vi "control.vi"(0 "tiempo (ms)":dbl, 5 "opticalPathMax (nm)":dbl, 7 "#samples":u32, 9 "lamda (nm)":dbl, 10 "SigmaMax (ms)":dbl, 12 "m":dbl, 13 "b":dbl) -> ()   [LabVIEW 2010]
panel:
  out "Prueba":dbl[](array[numeric])
  out "Final":dbl[](array[numeric])
  in  "queda?":bool=TRUE
  in  "delta t0 (ms)":dbl
  in  "Contraste":i32
  in  "Control?":bool
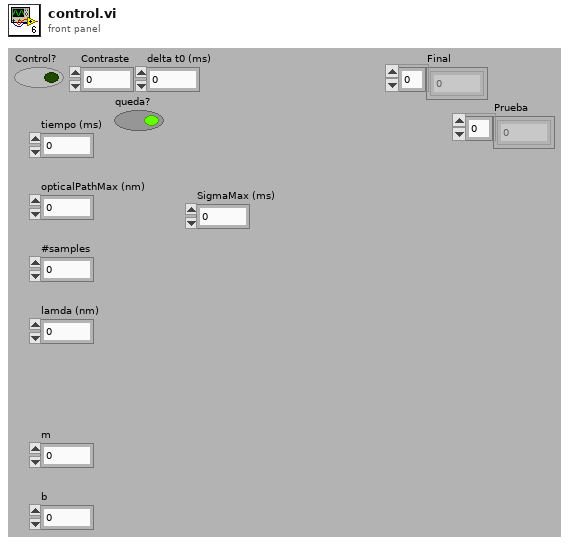
[diagram p1: front panel]
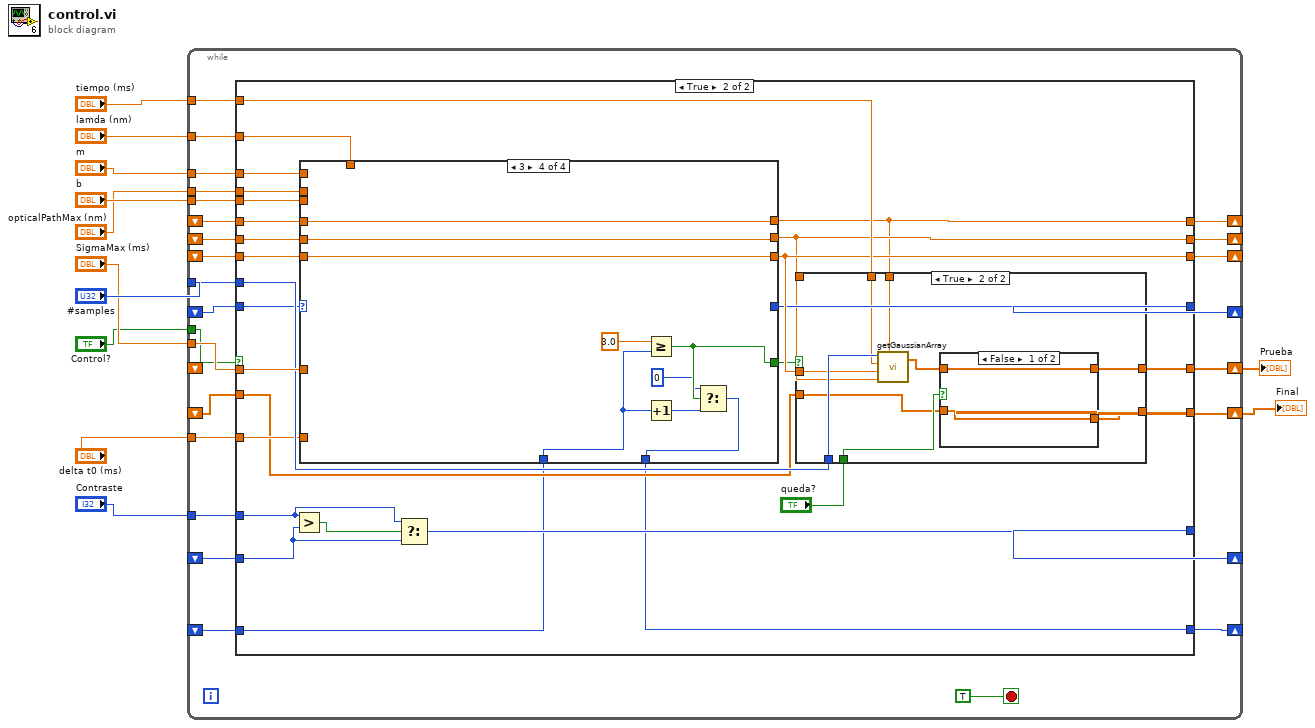
[diagram p0: block diagram]
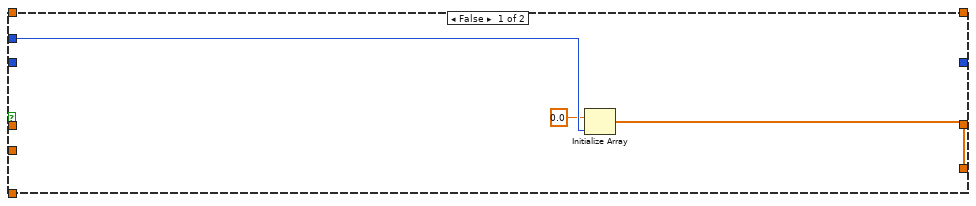
[diagram p2: hidden frame]
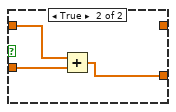
[diagram p4: hidden frame]
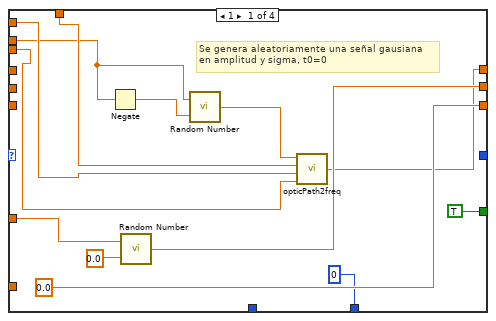
[diagram p5: hidden frame]
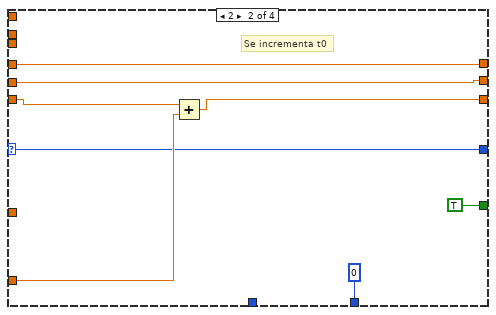
[diagram p6: hidden frame]
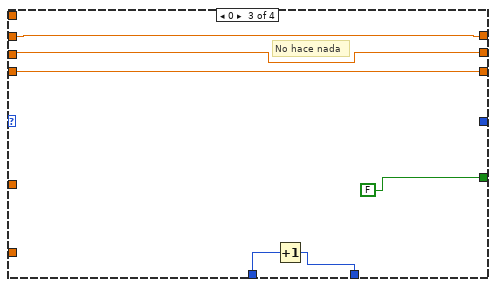
[diagram p7: hidden frame]
diagram:
  n1 = while {
    tunnel: "#samples" -> [w32]
    tunnel: "tiempo (ms)" -> [w31]
    shift-right: [w28] -> _
    shift-left: _ -> [w23]
    shift-right: [w29] -> _
    shift-left: _ -> [w22]
    shift-right: [w30] -> _
    shift-left: _ -> [w21]
    shift-right: [w17] -> _
    shift-left: _ -> [w18]
    tunnel: "lamda (nm)" -> [w37]
    tunnel: "m" -> [w36]
    tunnel: "b" -> [w35]
    tunnel: "SigmaMax (ms)" -> [w34]
    tunnel: "opticalPathMax (nm)" -> [w33]
    tunnel: "Contraste" -> [w26]
    shift-right: [w24] -> _
    shift-left: _ -> [w25]
    tunnel: "delta t0 (ms)" -> [w20]
    tunnel: "Control?" -> [w19]
    shift-right: [w27] -> w2
    shift-left: _ -> [w16]
    shift-right: [w15] -> w1
    shift-left: _ -> [_]
    shift-right: [w13] -> _
    shift-left: _ -> [w14]
    stop <- TRUE stop-if-true
    n2 = case shown="True" w19 {
      tunnel: w37 -> [_ w68]
      tunnel: w36 -> [_ w67]
      tunnel: w35 -> [_ w66]
      tunnel: w34 -> [_ w65]
      tunnel: w33 -> [_ w64]
      tunnel: w32 -> [w40 w63]
      tunnel: w31 -> [_ w62]
      tunnel: [_ w61] -> w30
      tunnel: [_ w60] -> w29
      tunnel: [_ w59] -> w28
      tunnel: [w41 w48] -> w27
      tunnel: w26 -> [_ w57]
      tunnel: w25 -> [_ w56]
      tunnel: [_ w55] -> w24
      tunnel: w23 -> [_ w54]
      tunnel: w22 -> [_ w53]
      tunnel: w21 -> [_ w52]
      tunnel: w20 -> [_ w51]
      tunnel: w18 -> [_ w50]
      tunnel: [_ w49] -> w17
      tunnel: w16 -> [_ w44]
      tunnel: [_ w46] -> w15
      tunnel: w14 -> [_ w42]
      tunnel: [_ w43] -> w13
      frame False {
        n3 = Initialize Array(0.0 ("element"), w40) -> (w41:dbl[])
      }
      frame True {
        n4 = Greater?(x=w57, y=w56) -> (0:w58:bool)
        n5 = case shown="3" w50 {
          selector: w50 -> [_ w100 _ _]
          tunnel: [w87 w105 w110 w119] -> w59
          tunnel: [w95 w104 w109 w118] -> w60
          tunnel: [0.0 ("t0 (ms)") w102 w108 w117] -> w61
          tunnel: w68 -> [w90 _ _ _]
          tunnel: w67 -> [w93 _ _ _]
          tunnel: w66 -> [w92 _ _ _]
          tunnel: w65 -> [w91 _ _ _]
          tunnel: w64 -> [w89 _ _ _]
          tunnel: w54 -> [_ w105 w110 w119]
          tunnel: w53 -> [_ w104 w109 w118]
          tunnel: w52 -> [_ w103 w108 w117]
          tunnel: w51 -> [_ w101 _ _]
          tunnel: [_ w100 _ _] -> w49
          tunnel: [TRUE TRUE FALSE w114] -> w45
          tunnel: [0 0 w106 w115] -> w43
          tunnel: w42 -> [_ _ w107 w116]
          frame 1 {
            # "Se genera aleatoriamente una señal gausiana \nen amplitud y sigma, t0=0"
            n6 = Negate(x=w89) -> (-x=w97:dbl)
            n7 = call "Random Number.vi"("Min"=0.0, "Max"=w91) -> ("Out"=w95:dbl)
            n8 = call "Random Number.vi"("Min"=w97, "Max"=w89) -> ("Out"=w88:dbl)
            n9 = call "opticPath2freq.vi"("b"=w92, "m"=w93, "lamda (nm)"=w90, "camino optico (nm)"=w88) -> ("freq"=w87:dbl)
          }
          frame 2 {
            # "Se incrementa t0"
            n10 = Add(x=w103, y=w101) -> (x+y=w102:dbl)
          }
          frame 0 {
            # "No hace nada"
            n11 = Increment(x=w107) -> (x+1=w106:i32)
          }
          frame 3 {
            n12 = Greater Or Equal?(x=3.0, y=w116) -> (x >= y?=w114:bool)
            n13 = Increment(x=w116) -> (x+1=w112:i32)
            n14 = Select(t=0 ("f"), s=w114, f=w112) -> (s? t:f=w115:i32)
          }
        }
        n15 = Select(t=w57, s=w58, f=w56) -> (s? t:f=w55:i32)
        n16 = case shown="True" w45 {
          tunnel: w63 -> [_ w79]
          tunnel: w62 -> [_ w78]
          tunnel: w61 -> [_ w77]
          tunnel: w60 -> [_ w76]
          tunnel: w59 -> [_ w75]
          tunnel: [w69 w71] -> w48
          tunnel: w44 -> [w69 w72]
          tunnel: "queda?" -> [_ w74]
          tunnel: [_ w70] -> w46
          frame False {
          }
          frame True {
            n17 = call "getGaussianArray.vi"("#samples"=w79, "tiempo (ms)"=w78, "t0 (ms)"=w77, "Sigma (ms)"=w76, "Amplitud"=w75) -> ("Y out"=w73:dbl[])  [unwired: 1 out]
            n18 = case shown="False" w74 {
              tunnel: w73 -> [w80 w84]
              tunnel: w72 -> [w81 w83]
              tunnel: [w81 w82] -> w71
              tunnel: [w80 _] -> w70
              frame False {
              }
              frame True {
                n19 = Add(x=w84, y=w83) -> (x+y=w82:dbl[])
              }
            }
          }
        }
      }
    }
  }
  "Final" <- w2
  "Prueba" <- w1
